vi "ArrSelCheck.vi"(8 "error in":errorcluster caption="错误输入", 11 "ArrayIn":string[](array[string])) -> (0 "error out":errorcluster caption="错误输出", 3 "Repeat?":bool)   [LabVIEW 2013]
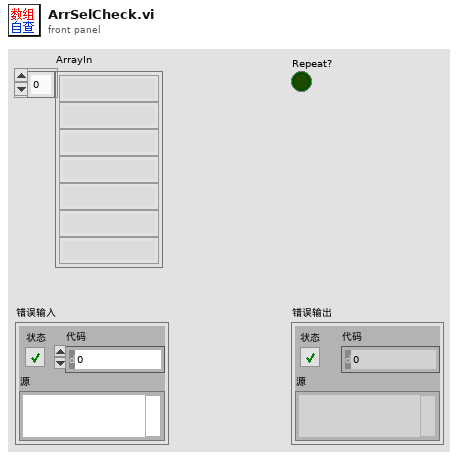
[diagram p1: front panel]
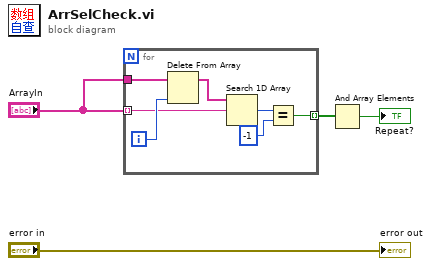
[diagram p0: block diagram]
diagram:
  n1 = for {
    tunnel: "ArrayIn" -> [w8] mode=indexing
    tunnel: "ArrayIn" -> [w11]
    tunnel: [w5] -> w3 mode=indexing
    i -> [w10]
    n2 = Delete From Array(array=w11, index=w10) -> (array with subset deleted=w9:string[])  [unwired: 1 in, 1 out]
    n3 = Search 1D Array(1D array=w9, element=w8) -> (index of element=w7:i32)  [unwired: 1 in]
    n4 = Equal?(x=w7, y=-1) -> (x = y?=w5:bool)
  }
  n5 = And Array Elements(Boolean array=w3) -> (logical AND=→"Repeat?":bool)
  "error out" <- "error in"
